vi "[FGV] ROI_List.vi"(4 "ROIEntriesIn":T1[](array[typedef]), 6 "ProcessSetting":T2[](array[typedef]), 7 "Action":T10, 8 "error in (no error)":errorcluster, 9 "ROIs_Index":i32[](array[numeric]), 10 "ROI_To_Add":T9, 11 "Analysis_Setting":T6={"PreProcess"=enum."*Algorithm*", "Parameter"=""}) -> (0 "error out":errorcluster, 1 "All ROI":T1[](array[typedef]), 2 "ROI Entry":T8={"vROIName"="", "vROIContour"={"Contour Type"=0, "ROI Type"=0, "Points"=[]}, "ProcessSetting"=[], "Analysis_Setting"={"PreProcess"=enum."*Algorithm*", "Parameter"=""}})   [LabVIEW 2019]
uses:
  Process/Controls/Process_Setting.ctl
  Analysis/Controls/Analysis_Setting.ctl
  Controls/Vision_DataEntry.ctl
  Analysis/Controls/V_Analysis_Type.ctl
  Ctrl/VisionProcessName.ctl
  Controls/ROI_List_Action.ctl
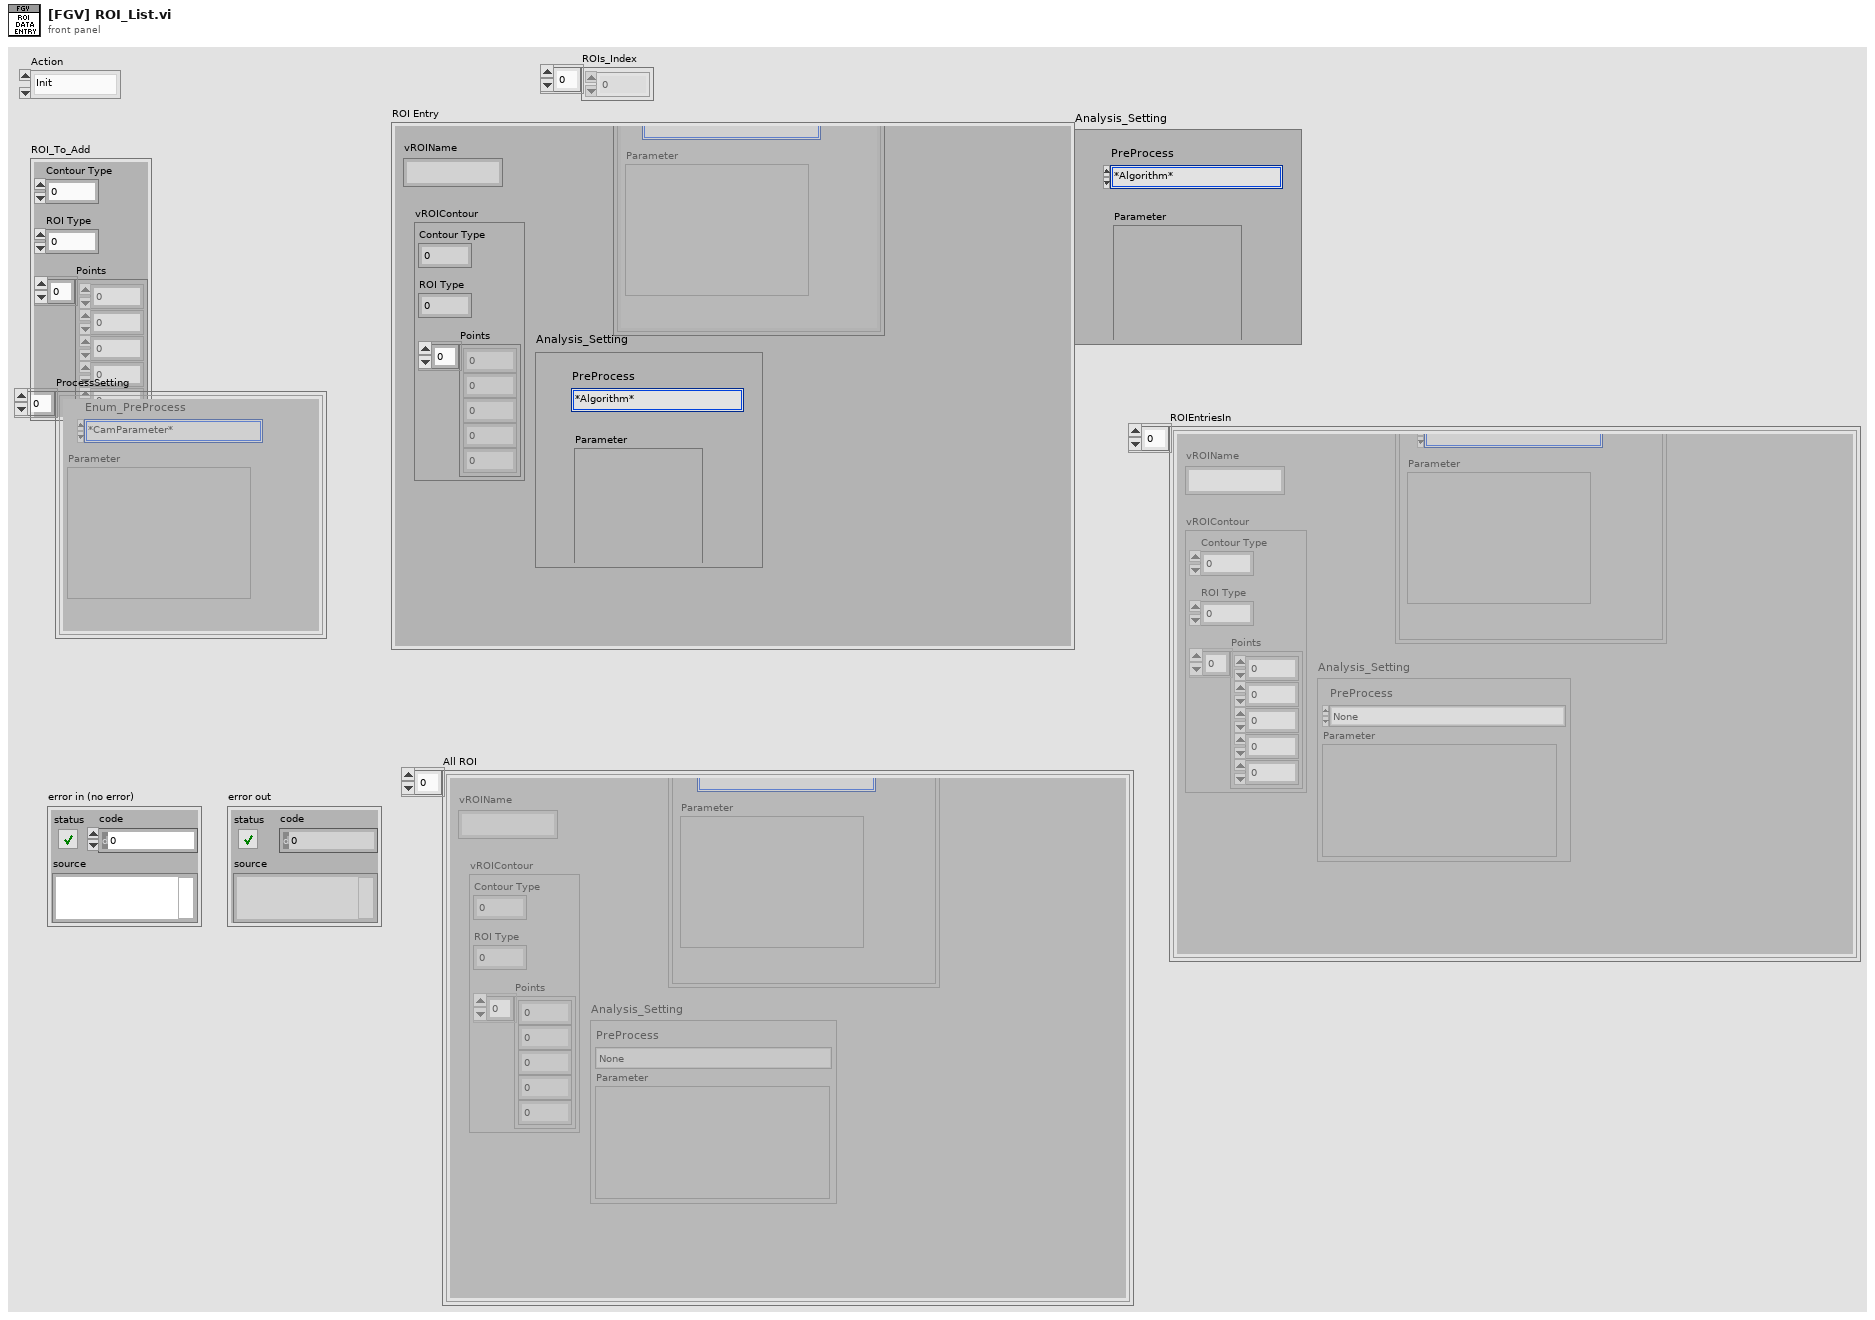
[diagram p1: front panel]
types:
  T1 = typedef "Vision_DataEntry.ctl" = cluster{"vROIName":string, "vROIContour":cluster{"Contour Type":u32, "ROI Type":u32, "Points":i32[]}, "ProcessSetting":T2[], "Analysis_Setting":T4}
  T2 = typedef "Process_Setting.ctl" = cluster{"Enum_PreProcess":T3, "Parameter":string}
  T3 = typedef "VisionProcessName.ctl" = enum16{"*CamParameter*", "CamAttributes", "*Preprocess*", "CG_Brightness", "C_Plane Extraction", "C_Threshold", "G_Lookup Table", "G_Threshold"}
  T4 = typedef "Analysis_Setting.ctl" = cluster{"PreProcess":T5, "Parameter":string}
  T5 = typedef "V_Analysis_Type.ctl" = enum16{"None", "C_Color Pattern Matching", "G_PatternMatching", "G_ShapeDectect", "G_GeometricMatch", "B_Area Check"}
  T6 = typedef "Analysis_Setting.ctl" = cluster{"PreProcess":T7, "Parameter":string}
  T7 = typedef "VisionProcessName.ctl" = enum16{"*CamParameter*", "CamAttributes", "*Preprocess*", "CG_Brightness", "C_Plane Extraction", "C_Threshold", "G_Lookup Table", "G_Threshold", "B_Image Inversion", "*Algorithm*", "CG_Histogram", "C_Color Matching", "C_Color Pattern Matching", "G_PatternMatch", "CG_Find Straight Edge", "CG_Adv. Find Straight Edge", "CG_Find Circular Edge", "G_Max Clamp", "G_Clamp (Rake)", "G_Pattern Matching"}
  T8 = typedef "Vision_DataEntry.ctl" = cluster{"vROIName":string, "vROIContour":cluster{"Contour Type":u32, "ROI Type":u32, "Points":i32[]}, "ProcessSetting":T2[], "Analysis_Setting":T6}
  T9 = cluster{"Contour Type":u32, "ROI Type":u32, "Points":i32[]}
  T10 = typedef "ROI_List_Action.ctl" = enum16{"Init", "Add ROI", "Delete ROI", "Get All ROI", "Get Specific ROI", "Set Analysis Setting", "Set Process Setting", "Replace All Entries", "ROIEntryBackup", "ROIEntryBackupClear", "ROIEntryReturn"}
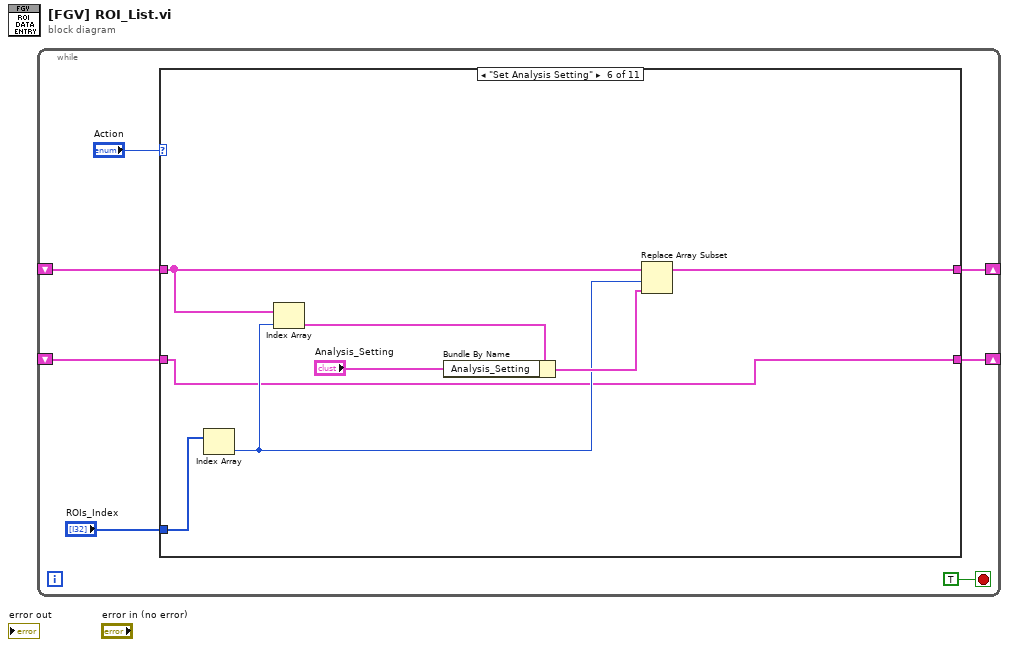
[diagram p0: block diagram]
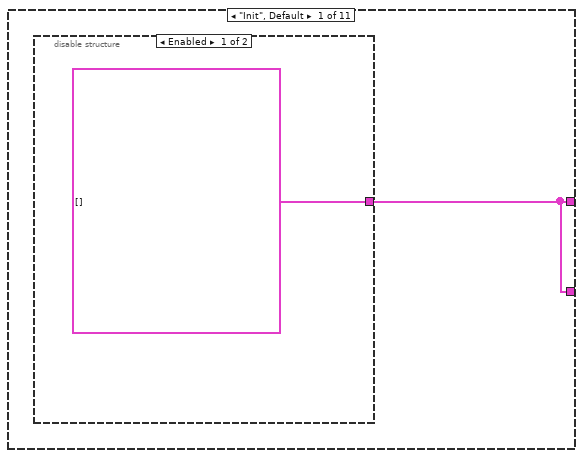
[diagram p2: hidden frame]
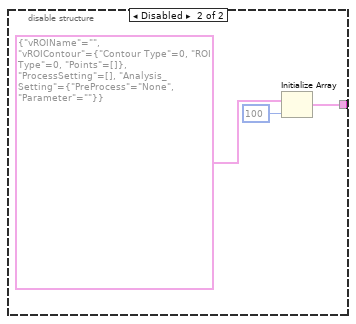
[diagram p3: hidden frame]
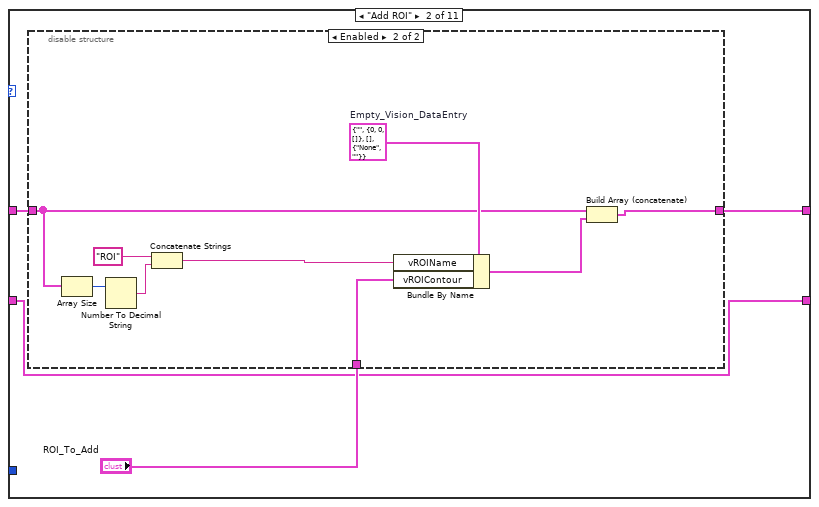
[diagram p4: hidden frame]
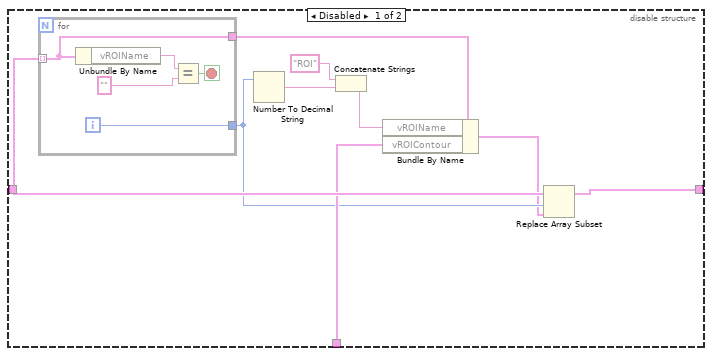
[diagram p5: hidden frame]
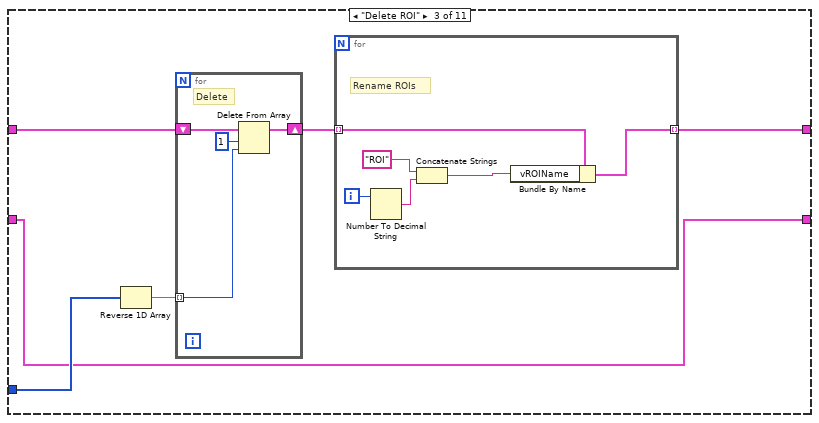
[diagram p6: hidden frame]
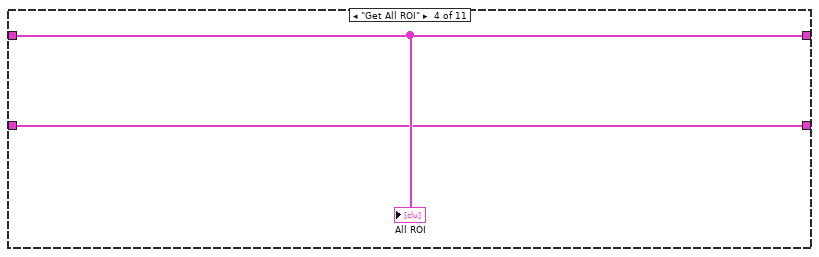
[diagram p7: hidden frame]
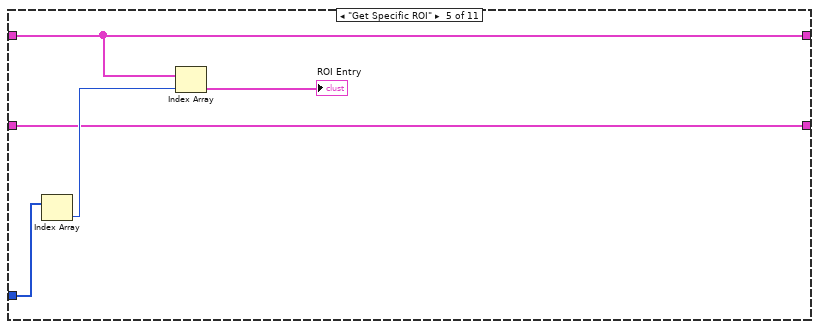
[diagram p8: hidden frame]
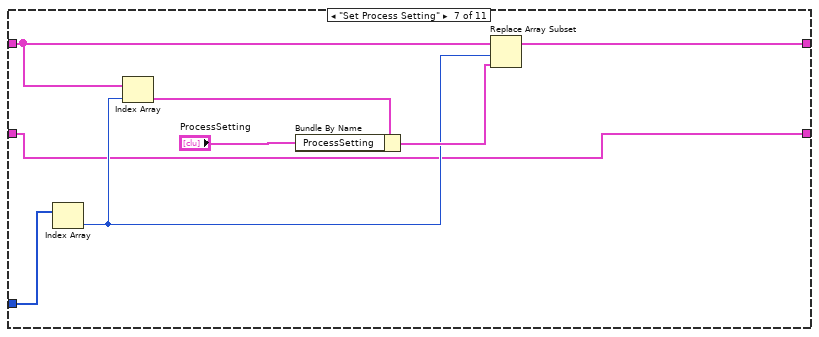
[diagram p9: hidden frame]
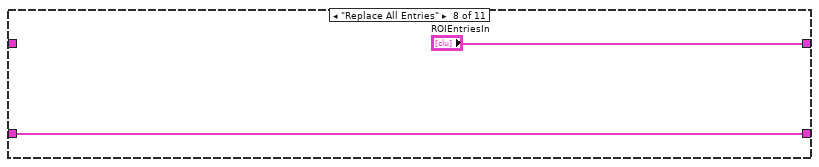
[diagram p10: hidden frame]
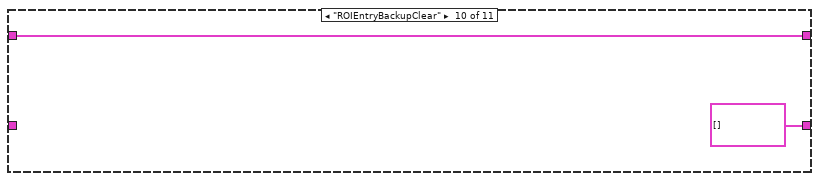
[diagram p12: hidden frame]
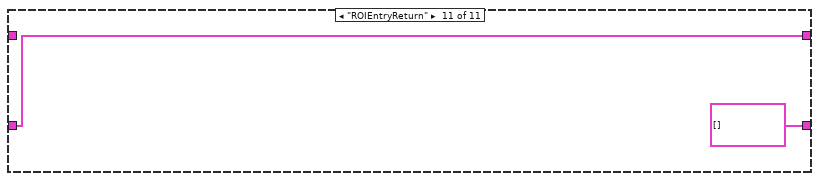
[diagram p13: hidden frame]
diagram:
  n1 = while {
    shift-right: [w5] -> _
    shift-left: _ -> [w4]
    shift-right: [w2] -> _
    shift-left: _ -> [w1]
    stop <- TRUE stop-if-true
    n2 = case shown="\"Set Analysis Setting\"" "Action" {
      tunnel: [w8 w16 w41 w57 w61 w65 w73 "ROIEntriesIn" w81 w83 w85] -> w5
      tunnel: w4 -> [_ w15 w45 w57 w61 w68 w76 _ w81 w83 _]
      tunnel: "ROIs_Index" -> [_ _ w44 _ w62 w70 w78 _ _ _ _]
      tunnel: [w8 w13 w40 w56 w58 w63 w71 w79 w81 T1[] [] ("ROIEntriesIn") T1[] [] ("ROIEntriesIn")] -> w2
      tunnel: w1 -> [_ w13 w40 w56 w58 w63 w71 w79 _ _ w85]
      frame "Init", Default {
        n3 = disable-structure shown="Enabled" {
          disable-tunnel: [T1[] [] w11] -> w8
          frame Enabled {
          }
          frame Disabled {
            n4 = Initialize Array(T1 {"vROIName"="", "vROIContour"={"Contour Type"=0, "ROI Type"=0, "Points"=[]}, "ProcessSetting"=[], "Analysis_Setting"={"PreProcess"=enum."None", "Parameter"=""}} ("Vision_DataEntry"), 100 ("dimension size")) -> (w11:T1[])
          }
        }
      }
      frame "Add ROI" {
        n5 = disable-structure shown="Enabled" {
          disable-tunnel: [w25 w32] -> w16
          disable-tunnel: w15 -> [w24 w34]
          disable-tunnel: "ROI_To_Add" -> [w22 w31]
          frame Disabled {
            n6 = for {
              tunnel: w24 -> [w27] mode=indexing
              tunnel: [w27] -> w23
              tunnel: [w26] -> w18
              i -> [w26]
              stop <- w28 stop-if-true
              n7 = Unbundle By Name(w27) -> ("vROIName"=w30:string)
              n8 = Equal?(x=w30, y="") -> (x = y?=w28:bool)
            }
            n9 = Number To Decimal String(number=w18) -> (decimal integer string=w21:string)  [unwired: 1 in]
            n10 = Concatenate Strings("ROI", w21) -> (w19:string)
            n11 = Bundle By Name(cluster=w23, "vROIName"=w19, "vROIContour"=w22) -> (w17:T1)
            n12 = Replace Array Subset(array=w24, new element=w17, index=w18) -> (w25:T1[])
          }
          frame Enabled {
            w36 = T1 {"vROIName"="", "vROIContour"={"Contour Type"=0, "ROI Type"=0, "Points"=[]}, "ProcessSetting"=[], "Analysis_Setting"={"PreProcess"=enum."None", "Parameter"=""}}  # Empty_Vision_DataEntry
            n13 = Array Size(array=w34) -> (size(s)=w39:i32)
            n14 = Number To Decimal String(number=w39) -> (decimal integer string=w37:string)  [unwired: 1 in]
            n15 = Concatenate Strings("ROI", w37) -> (w35:string)
            n16 = Bundle By Name(cluster=w36, "vROIName"=w35, "vROIContour"=w31) -> (w33:T1)
            n17 = Build Array (concatenate)(w34, w33) -> (w32:T1[])
          }
        }
      }
      frame "Delete ROI" {
        n18 = Reverse 1D Array(array=w44) -> (reversed array=w43:i32[])
        n19 = for {
          tunnel: w43 -> [w55] mode=indexing
          shift-right: [w53] -> w42
          shift-left: w45 -> [w54]
          # "Delete"
          n20 = Delete From Array(array=w54, length=1, index=w55) -> (array with subset deleted=w53:T1[])  [unwired: 1 out]
        }
        n21 = for {
          tunnel: w42 -> [w48] mode=indexing
          tunnel: [w46] -> w41 mode=indexing
          i -> [w51]
          # "Rename ROIs"
          n22 = Number To Decimal String(number=w51) -> (decimal integer string=w49:string)  [unwired: 1 in]
          n23 = Concatenate Strings("ROI", w49) -> (w47:string)
          n24 = Bundle By Name(cluster=w48, "vROIName"=w47) -> (w46:T1)
        }
      }
      frame "Get All ROI" {
        "All ROI" <- w57
      }
      frame "Get Specific ROI" {
        n25 = Index Array(array=w62) -> (element=w60:i32)  [unwired: 1 in]
        n26 = Index Array(array=w61, index=w60) -> (element=→"ROI Entry":T1)
      }
      frame "Set Analysis Setting" {
        n27 = Index Array(array=w70) -> (element=w66:i32)  [unwired: 1 in]
        n28 = Index Array(array=w68, index=w66) -> (element=w69:T1)
        n29 = Bundle By Name(cluster=w69, "Analysis_Setting"="Analysis_Setting") -> (w67:T1)
        n30 = Replace Array Subset(array=w68, new element=w67, index=w66) -> (w65:T1[])
      }
      frame "Set Process Setting" {
        n31 = Index Array(array=w78) -> (element=w74:i32)  [unwired: 1 in]
        n32 = Index Array(array=w76, index=w74) -> (element=w77:T1)
        n33 = Bundle By Name(cluster=w77, "ProcessSetting"="ProcessSetting") -> (w75:T1)
        n34 = Replace Array Subset(array=w76, new element=w75, index=w74) -> (w73:T1[])
      }
      frame "Replace All Entries" {
      }
      frame "ROIEntryBackup" {
      }
      frame "ROIEntryBackupClear" {
      }
      frame "ROIEntryReturn" {
      }
    }
  }
